vi "system off.vi"() -> ()   [LabVIEW 2009]
panel:
  out "dup VISA session":refnum<visa-resource-name>
  in  "VISA session":refnum<visa-resource-name>
  out "error out":errorcluster
  in  "error in (no error)":errorcluster
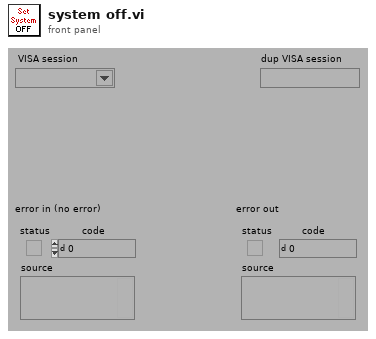
[diagram p1: front panel]
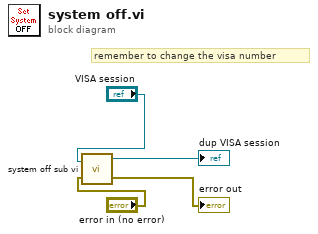
[diagram p0: block diagram]
diagram:
  # "remember to change the visa number"
  n1 = call "system off sub vi.vi"("error in (no error)"="error in (no error)", "VISA session"="VISA session") -> ("error out"=→"error out":errorcluster, "dup VISA session"=→"dup VISA session":refnum<visa-resource-name>)
